vi "Drive Convert relative position to absolute position.vi"(6 "Right Encoder position":i32, 9 "Left Encoder Position":i32, 10 "Timestamp [ms]":dbl, 11 "Relative Distance change":dbl) -> (2 "Right Target Position":dbl, 3 "Left Target Position":dbl)   [LabVIEW 2019]
uses:
  d62ed10b-4951-4d1f-aec3-b06ba0bdeac0.vi
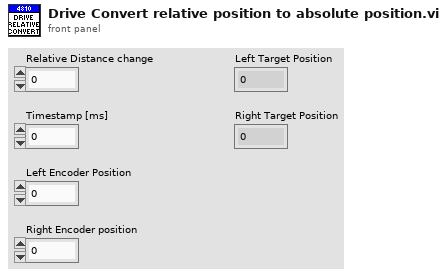
[diagram p1: front panel]
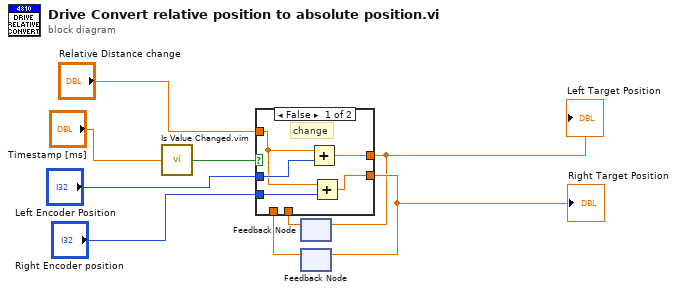
[diagram p0: block diagram]
diagram:
  n1 = call "Is Value Changed.vim"("value"="Timestamp [ms]") -> ("changed or first call?"=w1:bool)
  n2 = feedback #1() -> (w7:dbl)  [unwired: 1 in]
  n3 = feedback #2() -> (w9:dbl)  [unwired: 1 in]
  n4 = case shown="False" w1 {
    tunnel: "Relative Distance change" -> [w13 _]
    tunnel: "Left Encoder Position" -> [w14 _]
    tunnel: "Right Encoder position" -> [w12 _]
    tunnel: [w11 w16] -> w6
    tunnel: [w10 w15] -> w8
    tunnel: w7 -> [_ w16]
    tunnel: w9 -> [_ w15]
    frame False {
      # "change"
      n5 = Add(x=w13, y=w14) -> (x+y=w11:dbl)
      n6 = Add(x=w13, y=w12) -> (x+y=w10:dbl)
    }
    frame True {
      # "no change"
    }
  }
  "Right Target Position" <- w8
  "Left Target Position" <- w6
  n7 = feedback-in #1(w6) -> ()
  n8 = feedback-in #2(w8) -> ()
